vi "onGetPlatanoVarietal.vi"(8 "error in (no error)":errorcluster, 11 "Platano in":refnum<class "Platano.lvclass">) -> (0 "error out":errorcluster, 2 "Varietal":string, 3 "Platano out":refnum<class "Platano.lvclass">)   [LabVIEW 2021, in "Bananas.lvlib" / "Platano.lvclass"]
uses:
  Platano.lvclass
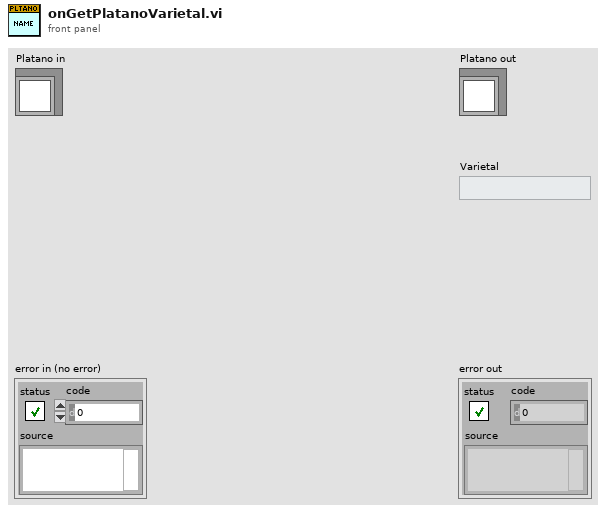
[diagram p1: front panel]
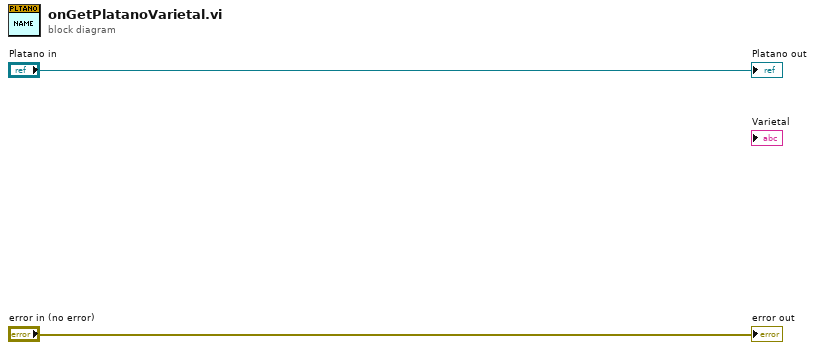
[diagram p0: block diagram]
diagram:
  "error out" <- "error in (no error)"
  "Platano out" <- "Platano in"
